vi "Get Parameter Scaling.vi"(8 "error in (no error)":errorcluster, 11 "Item Ref in":T1 format="%.0x") -> (0 "error out":errorcluster, 1 "scale offset":dbl, 2 "scale multiplier":dbl, 3 "Item Ref out":T1 format="%.0x")   [LabVIEW 2020, in "Communication Bus Template Scripting.lvlib"]
uses:
  Communication Bus Template Scripting.lvlib
  <vilib>/NI VeriStand/Custom Device API/Custom Device API.lvlib
  <vilib>/NI VeriStand/Custom Device API/Get Item Property (Double).vi
  Constants.vi
  <vilib>/NI VeriStand/Custom Device API/Custom Device Item Ref.ctl
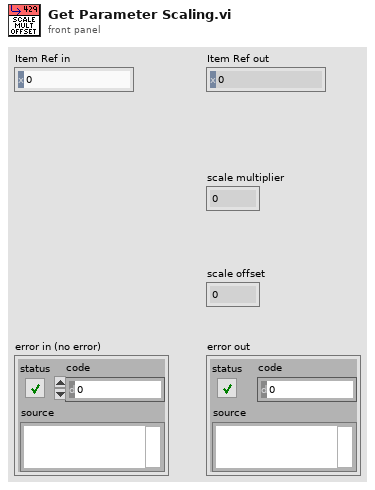
[diagram p1: front panel]
types:
  T1 = typedef "Custom Device API.lvlib/Custom Device Item Ref.ctl" = u64
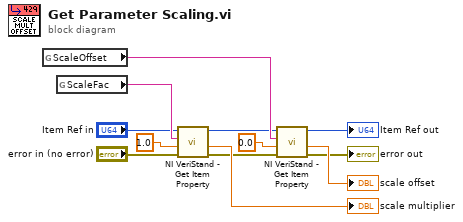
[diagram p0: block diagram]
diagram:
  n1 = global read "Constants.vi" "ScaleOffset"() -> (w8:string)
  n2 = global read "Constants.vi" "ScaleFac"() -> (w7:string)
  n3 = call-poly <vilib>:"NI VeriStand - Get Item Property.vi"("error in (no error)"="error in (no error)", "Default Value"=1.0, "Property Name"=w7, "Item Ref in"="Item Ref in") -> ("error out"=w4:errorcluster, "Value"=→"scale multiplier":dbl, "Item Ref out"=w1:T1)  [unwired: 4 in, 1 out]
  n4 = call-poly <vilib>:"NI VeriStand - Get Item Property.vi"("error in (no error)"=w4, "Default Value"=0.0, "Property Name"=w8, "Item Ref in"=w1) -> ("error out"=→"error out":errorcluster, "Value"=→"scale offset":dbl, "Item Ref out"=→"Item Ref out":T1)  [unwired: 4 in, 1 out]
